vi "displayChannelList.vi"(8 "error in (no error)":errorcluster, 11 "StaticOutputEditor in":refnum<class "StaticOutputEditor.lvclass">) -> (0 "error out":errorcluster, 3 "StaticOutputEditor out":refnum<class "StaticOutputEditor.lvclass">)   [LabVIEW 2011, in "Views.lvlib" / "ScriptEditor.lvlib" / "StaticOutputEditor.lvclass"]
uses:
  StaticOutputEditor.lvclass
  StaticOutputEditor.lvclass/StaticOutputEditor.ctl
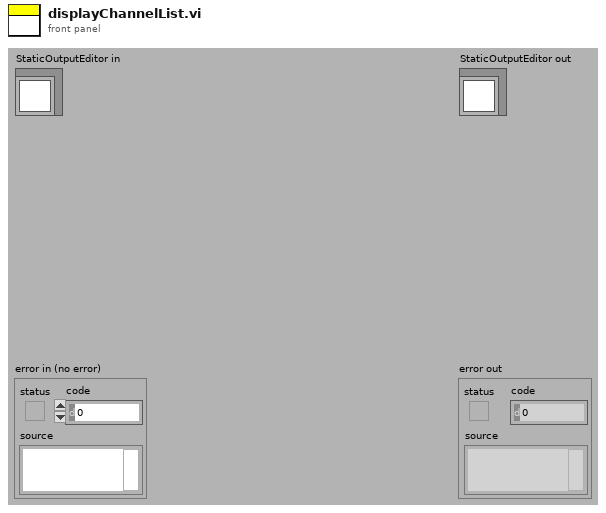
[diagram p1: front panel]
types:
  T1 = cluster{"channel":string, string, string, string}
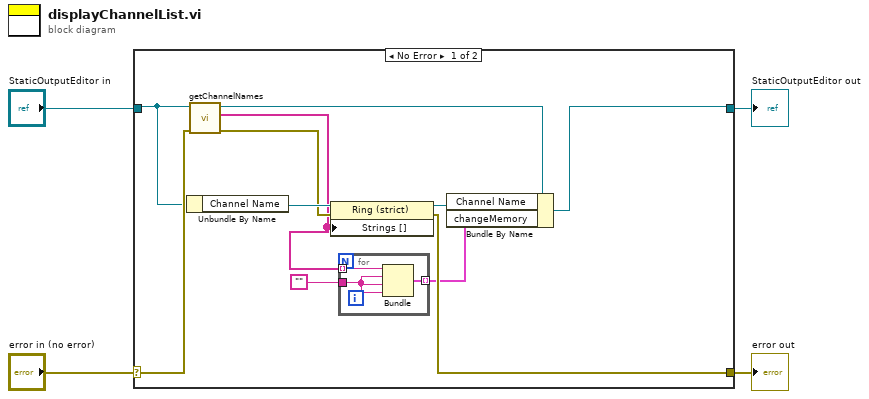
[diagram p0: block diagram]
diagram:
  n1 = case shown="No Error" "error in (no error)" {
    selector: "error in (no error)" -> [w15 w20]
    tunnel: [w8 w20] -> w3
    tunnel: [w9 w19] -> w1
    tunnel: "StaticOutputEditor in" -> [w14 w19]
    frame No Error {
      n2 = Unbundle By Name(w14) -> ("Channel Name"=w13:refnum<vi>)
      n3 = call "getChannelNames.vi"("error in (no error)"=w15, "StaticOutputEditor in"=w14) -> ("error out"=w12:errorcluster, "channelNames"=w7:string[], "StaticOutputEditor out"=w10:refnum<class "StaticOutputEditor.lvclass">)  [unwired: 7 in]
      n4 = property class="Ring (strict)"(reference=w13, error in=w12, "Strings []"=w7) -> (reference out=w11:refnum<vi>, error out=w8:errorcluster)
      n5 = for {
        tunnel: w7 -> [w18] mode=indexing
        tunnel: "" -> [w17]
        tunnel: [w16] -> w5 mode=indexing
        n6 = Bundle("channel"=w18, w17, w17, w17) -> (w16:T1)  [unwired: 1 in]
      }
      n7 = Bundle By Name(cluster=w10, "Channel Name"=w11, "changeMemory"=w5) -> (w9:refnum<class "StaticOutputEditor.lvclass">)
    }
    frame Error {
    }
  }
  "error out" <- w3
  "StaticOutputEditor out" <- w1
